vi "Init_UI_Start.vi"(8 "error in (no error)":errorcluster, 11 "Cluster_IN":T1) -> (0 "error out":errorcluster, 3 "Cluster_OUT":T1)   [LabVIEW 2020]
uses:
  Controls/UI_Cluster.ctl
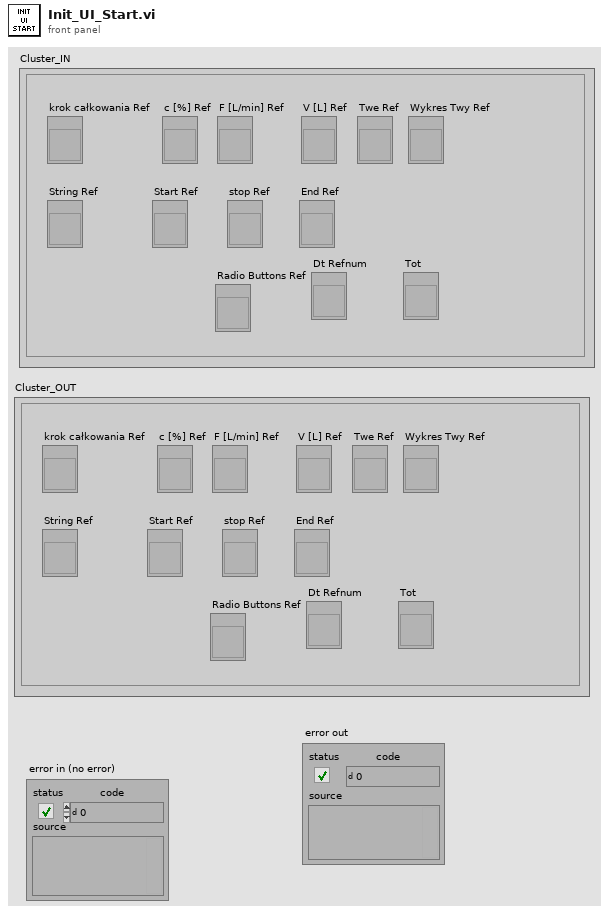
[diagram p1: front panel]
types:
  T1 = typedef "UI_Cluster.ctl" = cluster{"krok całkowania Ref":refnum<vi>, "c [%] Ref":refnum<vi>, "F [L/min] Ref":refnum<vi>, "V [L] Ref":refnum<vi>, "Twe Ref":refnum<vi>, "Wykres Twy Ref":refnum<vi>, "String Ref":refnum<vi>, "Start Ref":refnum<vi>, "stop Ref":refnum<vi>, "End Ref":refnum<vi>, "Dt Refnum":refnum<vi>, "Radio Buttons Ref":refnum<vi>, "Tot":refnum<vi>}
  T2 = enum8{"Enabled", "Disabled", "Disabled and Grayed Out"}
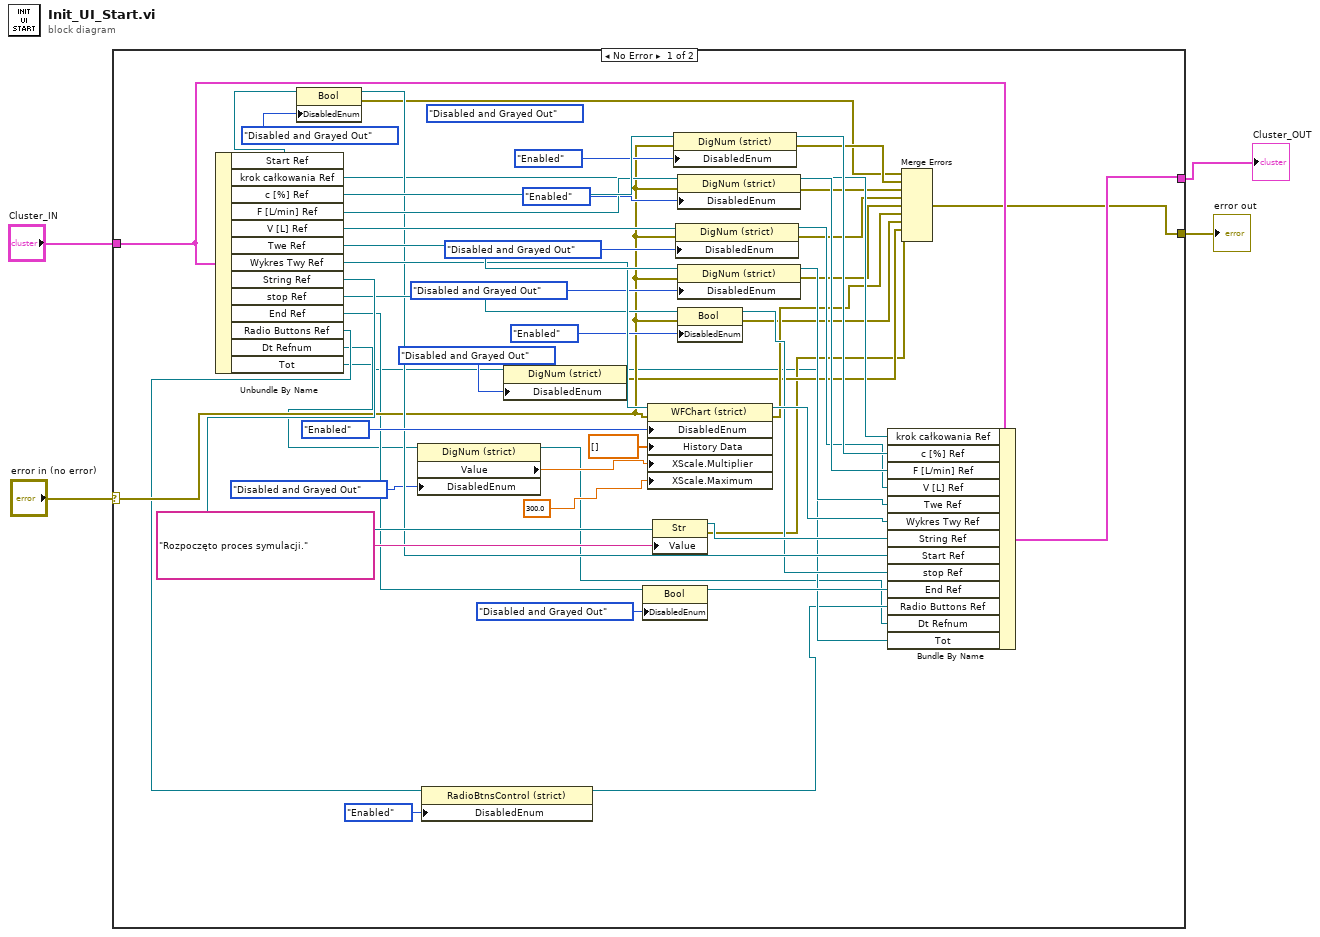
[diagram p0: block diagram]
diagram:
  n1 = case shown="No Error" "error in (no error)" {
    selector: "error in (no error)" -> [w30 w58]
    tunnel: "Cluster_IN" -> [w53 w59]
    tunnel: [w44 w59] -> w2
    tunnel: [w43 w58] -> w1
    frame No Error {
      (unwired) T2."Disabled and Grayed Out" ("Disabled")
      n2 = Unbundle By Name(w53) -> ("Start Ref"=w36:refnum<vi>, "krok całkowania Ref"=w24:refnum<vi>, "c [%] Ref"=w57:refnum<vi>, "F [L/min] Ref"=w51:refnum<vi>, "V [L] Ref"=w55:refnum<vi>, "Twe Ref"=w54:refnum<vi>, "Wykres Twy Ref"=w47:refnum<vi>, "String Ref"=w42:refnum<vi>, "stop Ref"=w34:refnum<vi>, "End Ref"=w29:refnum<vi>, "Radio Buttons Ref"=w7:refnum<vi>, "Dt Refnum"=w6:refnum<vi>, "Tot"=w5:refnum<vi>)
      n3 = property class="Bool"(reference=w36, "DisabledEnum"=T2."Disabled and Grayed Out" ("Disabled")) -> (reference out=w32:refnum<vi>, error out=w13:errorcluster)  [unwired: 1 in]
      n4 = property class="DigNum (strict)"(reference=w6, "DisabledEnum"=T2."Disabled and Grayed Out" ("Disabled")) -> (reference out=w8:refnum<vi>, "Value"=w17:dbl)  [unwired: 1 in, 1 out]
      n5 = property class="RadioBtnsControl (strict)"(reference=w7, "DisabledEnum"=T2."Enabled" ("Disabled")) -> (reference out=w9:refnum<vi>)  [unwired: 1 in, 1 out]
      n6 = property class="DigNum (strict)"(reference=w5, "DisabledEnum"=T2."Disabled and Grayed Out" ("Disabled")) -> (reference out=w10:refnum<vi>, error out=w12:errorcluster)  [unwired: 1 in]
      n7 = property class="Bool"(reference=w29, "DisabledEnum"=T2."Disabled and Grayed Out" ("Disabled")) -> (reference out=w27:refnum<vi>)  [unwired: 1 in, 1 out]
      n8 = property class="WFChart (strict)"(reference=w47, error in=w30, "DisabledEnum"=T2."Enabled" ("Disabled"), "History Data"=dbl[] [], "XScale.Multiplier"=w17, "XScale.Maximum"=300.0 ("f")) -> (reference out=w45:refnum<vi>, error out=w19:errorcluster)
      n9 = property class="Str"(reference=w42, "Value"="Rozpoczęto proces symulacji.") -> (reference out=w40:refnum<vi>, error out=w11:errorcluster)  [unwired: 1 in]
      n10 = property class="DigNum (strict)"(reference=w57, error in=w30, "DisabledEnum"=T2."Enabled" ("Disabled")) -> (reference out=w52:refnum<vi>, error out=w23:errorcluster)
      n11 = property class="DigNum (strict)"(reference=w55, error in=w30, "DisabledEnum"=T2."Disabled and Grayed Out" ("Disabled")) -> (reference out=w49:refnum<vi>, error out=w21:errorcluster)
      n12 = property class="DigNum (strict)"(reference=w51, error in=w30, "DisabledEnum"=T2."Enabled" ("Disabled")) -> (reference out=w50:refnum<vi>, error out=w22:errorcluster)
      n13 = property class="DigNum (strict)"(reference=w54, error in=w30, "DisabledEnum"=T2."Disabled and Grayed Out" ("Disabled")) -> (reference out=w48:refnum<vi>, error out=w20:errorcluster)
      n14 = property class="Bool"(reference=w34, error in=w30, "DisabledEnum"=T2."Enabled" ("Disabled")) -> (reference out=w31:refnum<vi>, error out=w18:errorcluster)
      n15 = Bundle By Name(cluster=w53, "krok całkowania Ref"=w24, "c [%] Ref"=w52, "F [L/min] Ref"=w50, "V [L] Ref"=w49, "Twe Ref"=w48, "Wykres Twy Ref"=w45, "String Ref"=w40, "Start Ref"=w32, "stop Ref"=w31, "End Ref"=w27, "Radio Buttons Ref"=w9, "Dt Refnum"=w8, "Tot"=w10) -> (w44:T1)
      n16 = Merge Errors(w13, w23, w22, w21, w20, w19, w18, w12, w11) -> (w43:errorcluster)
    }
    frame Error {
    }
  }
  "Cluster_OUT" <- w2
  "error out" <- w1
